vi "Start Module.vi"(6 "Show Main VI Diagram on Init (F)":bool, 7 "Panel":refnum<class "Panel.lvclass"> caption="Panel (Window)", 8 "error in (no error)":errorcluster) -> (0 "error out":errorcluster, 1 "Wait for Event Sync?":bool, 2 "Chart Broadcast Events":T1, 3 "Module Was Already Running?":bool, 4 "Module Name":string)   [LabVIEW 2024, in "Chart.lvlib"]
doc: "Launches the Module Main.vi.\n_____\nCreated using DQMH Event Scripter 6.0.0.122.\n\n<b>Note:</b> This VI was modified by the <b>Validate DQMH Module</b> tool to add calls to the Semaphore VIs to synchronize actions between the Start Module and Stop Module VIs.\n\n<b>Note:</b> This VI was modified by the <b>Validate DQMH Module</b> tool to add the 'Show Main VI Diagram on Init' functionality included in DQMH 6.1.\n\nThe <b>Validate DQMH Module</b> tool added a 'Module Name' output to this VI."
uses:
  Chart.lvlib
  Broadcast Events--cluster.ctl
  Did Init Argument--cluster.ctl
  Status Updated Argument--cluster.ctl
  Error Reported Argument--cluster.ctl
  Stop Argument--cluster.ctl
  Get Module Execution Status Argument--cluster.ctl
  <vilib>/MGI/Panel Manager/Panel/Panel/Panel.lvclass
  <vilib>/Delacor/Delacor QMH/Libraries/Module Admin_class/Delacor_lib_QMH_Module Admin.lvclass
  <vilib>/Delacor/Delacor QMH/Libraries/Module Admin_class/Delacor_lib_QMH_Module Admin.lvclass/Delacor_lib_QMH_Module Admin.ctl
  <vilib>/Delacor/Delacor QMH/Libraries/Module Admin_class/Delacor_lib_QMH_Set External Launch.vi
  <vilib>/MGI/Panel Manager/Panel/Panel/Window/Window.lvclass
  C:/Program Files/National Instruments/LabVIEW 2025/vi.lib/MGI/Panel Manager/Panel/Panel/Panel.lvclass
  <vilib>/MGI/Panel Manager/Panel/Panel/Window/Window.vi
  <vilib>/Utility/error.llb/Error Cluster From Error Code.vi
  <vilib>/ErrorRing/Error Ring.xnode
  <vilib>/MGI/Panel Manager/Panel/Panel.lvlib
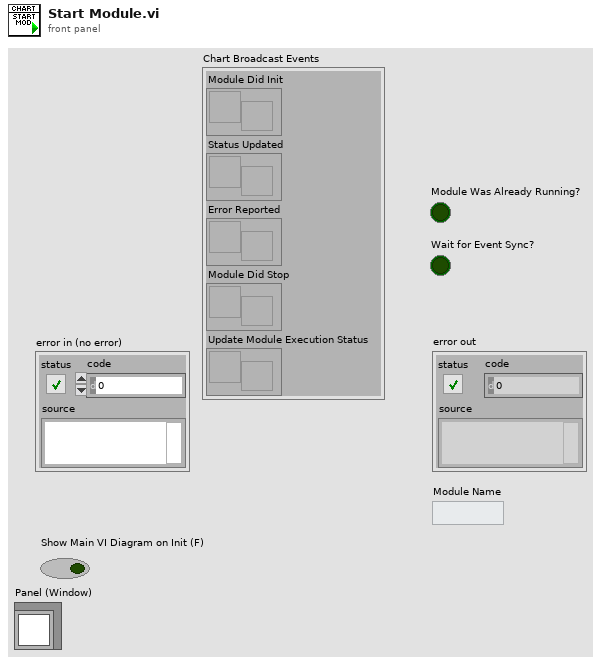
[diagram p1: front panel]
types:
  T1 = typedef "Chart.lvlib/Broadcast Events--cluster.ctl" = cluster{"Module Did Init":refnum<user-event>, "Status Updated":refnum<user-event>, "Error Reported":refnum<user-event>, "Module Did Stop":refnum<user-event>, "Update Module Execution Status":refnum<user-event>}
  T2 = enum32{"Bad", "Idle", "Run top level", "Running"}
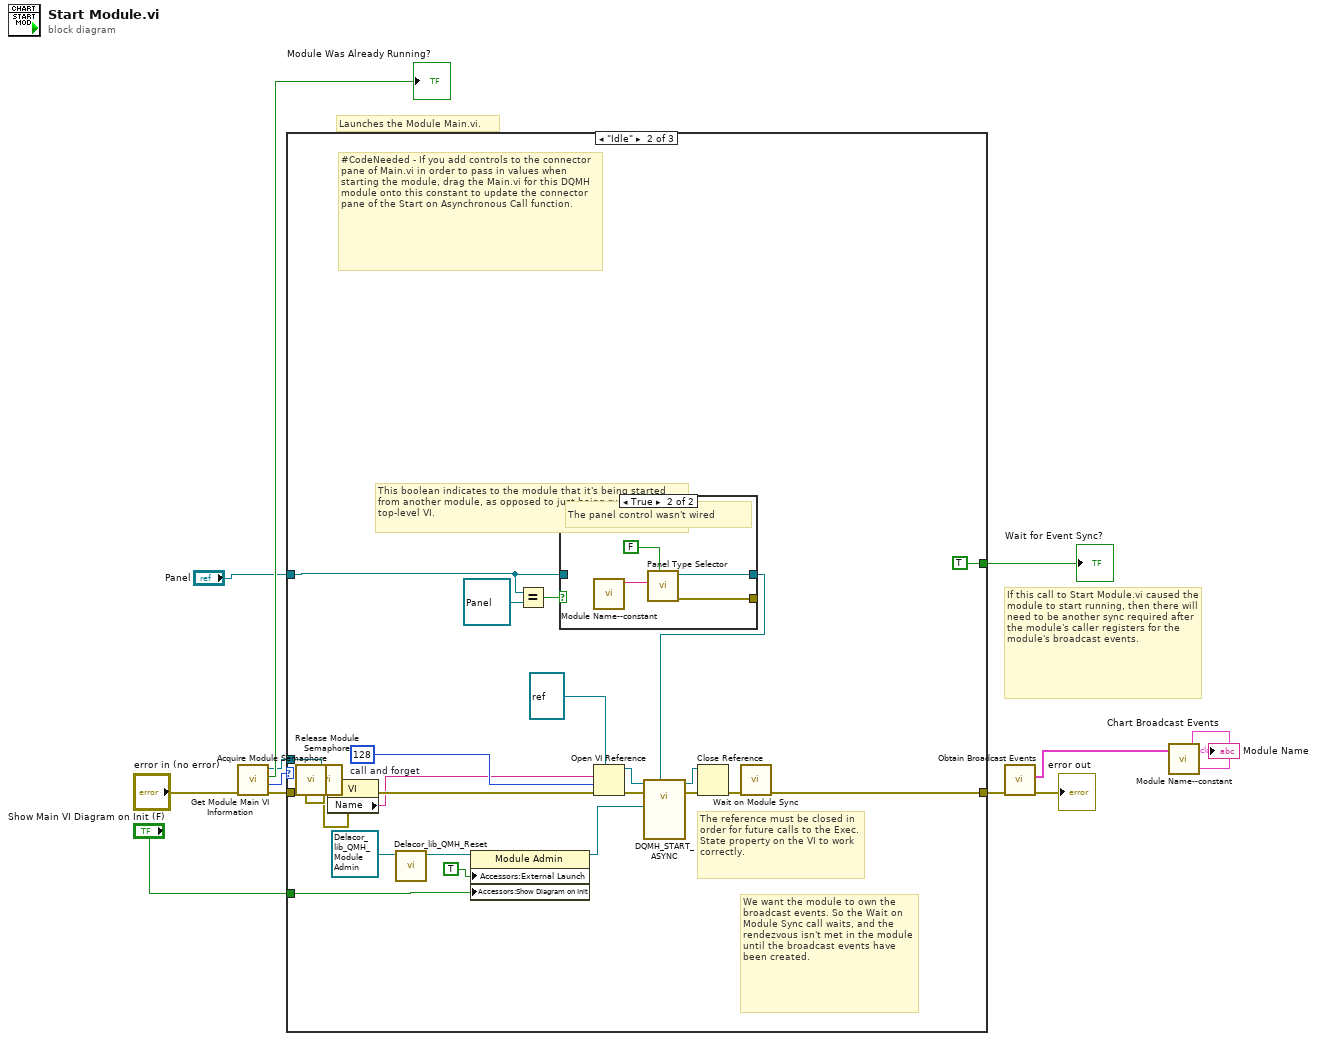
[diagram p0: block diagram]
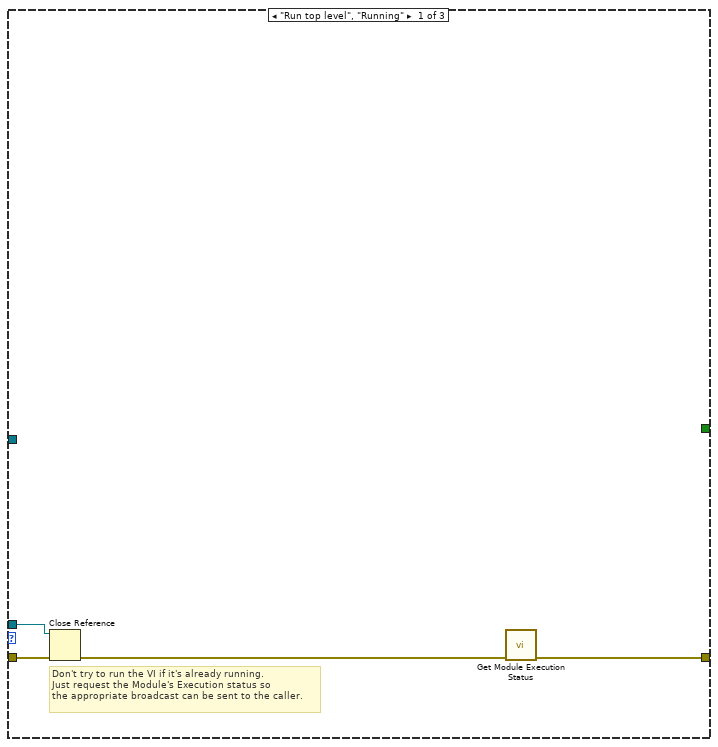
[diagram p2: hidden frame]
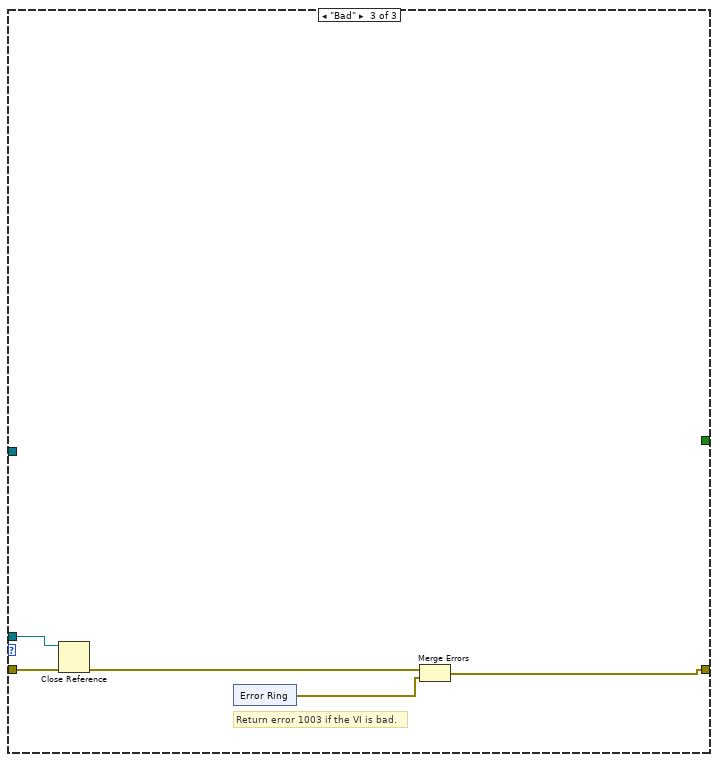
[diagram p4: hidden frame]
diagram:
  # "If this call to Start Module.vi caused the module to start running, then there will need to be another sync required after the module's caller registers for the module's broadcast events."
  # "Launches the Module Main.vi."
  n1 = call "Get Module Main VI Information.vi"("error in (no error)"="error in (no error)") -> ("error out"=w10:errorcluster, "Execution State"=w9:T2, "Is Module Running?"=→"Module Was Already Running?":bool, "Module Main VI"=w7:refnum<vi>)  [unwired: 7 in]
  n2 = case shown="\"Idle\"" w9 {
    tunnel: w10 -> [w16 w40 w50]
    tunnel: w7 -> [w15 w35 w49]
    tunnel: [w13 w25 w47] -> w6
    tunnel: [_ TRUE _] -> w12
    tunnel: "Panel" -> [_ w21 _]
    tunnel: "Show Main VI Diagram on Init (F)" -> [_ w17 _]
    frame "Run top level", "Running" {
      # "Don't try to run the VI if it's already running.\nJust request the Module's Execution status so\nthe appropriate broadcast can be sent to the caller."
      n3 = Close Reference(reference=w15, error in (no error)=w16) -> (error out=w14:errorcluster)
      n4 = call "Get Module Execution Status.vi"("error in (no error)"=w14) -> ("error out"=w13:errorcluster)  [unwired: 10 in]
    }
    frame "Idle" {
      w32 = 128  # call and forget
      # "#CodeNeeded - If you add controls to the connector pane of Main.vi in order to pass in values when starting the module, drag the Main.vi for this DQMH module onto this constant to update the connector pane of the Start on Asynchronous Call function."
      # "The reference must be closed in order for future calls to the Exec.State property on the VI to work correctly."
      # "We want the module to own the broadcast events. So the Wait on Module Sync call waits, and the rendezvous isn't met in the module until the broadcast events have been created."
      # "This boolean indicates to the module that it's being started from another module, as opposed to just being run as a top-level VI."
      n5 = call "Acquire Module Semaphore.vi"("error in"=w40) -> ("error out"=w19:errorcluster)  [unwired: 10 in]
      n6 = call "Release Module Semaphore.vi"("error in"=w19) -> ("error out"=w18:errorcluster)  [unwired: 10 in]
      n7 = property class="VI"(reference=w35, error in=w18) -> (error out=w34:errorcluster, "Name"=w27:string)  [unwired: 1 out]
      n8 = call-dynamic "Delacor_lib_QMH_Reset.vi"("Mod Admin in"=refnum<class "Delacor_lib_QMH_Module Admin.lvclass"> refnum) -> ("Mod Admin out"=w38:refnum<class "Delacor_lib_QMH_Module Admin.lvclass">)  [unwired: 9 in, 1 out]
      n9 = property on="DQMH_ADMIN_PROP_NODE" class="Module Admin"(reference=w38, "Accessors:External Launch"=TRUE ("DQMH_EXTERNAL_LAUNCH"), "Accessors:Show Diagram on Init"=w17) -> (reference out=w24:refnum<class "Delacor_lib_QMH_Module Admin.lvclass">)  [unwired: 1 in, 1 out]
      n10 = Equal?(x=w21, y=refnum<class "Panel.lvclass"> refnum) -> (x = y?=w22:bool)
      n11 = case shown="True" w22 {
        tunnel: w21 -> [w41 _]
        tunnel: [w41 w45] -> w20
        tunnel: [_ w42] -> _
        frame False {
          # "A panel object was wired in."
        }
        frame True {
          # "The panel control wasn't wired"
          n12 = call "Module Name--constant.vi"() -> ("Module Name"=w43:string)  [unwired: 11 in]
          n13 = call-poly <vilib>:"Panel Type Selector.vi"("Autoshow? (T)"=FALSE, "Default Title"=w43) -> ("error out"=w42:errorcluster, "Window out"=w45:refnum<class "Window.lvclass">)  [unwired: 8 in]
        }
      }
      n14 = Open VI Reference(type specifier VI Refnum (for type only)=refnum<vi> refnum ("DQMH_TYPE_SPECIFIER"), vi path=w27, options=w32, error in (no error)=w34) -> (vi reference=w30:refnum<vi>, error out=w31:errorcluster)  [unwired: 2 in]
      n15 = call-by-ref "DQMH_START_ASYNC"(reference=w30, error in=w31, "Panel"=w20, "Module Admin"=w24) -> (reference out=w28:refnum<vi>, error out=w29:errorcluster)  [unwired: 10 in]
      n16 = Close Reference ("DQMH_CLOSE_REF")(reference=w28, error in (no error)=w29) -> (error out=w26:errorcluster)
      n17 = call "Wait on Module Sync.vi"("error in (no error)"=w26) -> ("error out"=w25:errorcluster)  [unwired: 10 in]
    }
    frame "Bad" {
      # "Return error 1003 if the VI is bad."
      n18 = Close Reference(reference=w49, error in (no error)=w50) -> (error out=w48:errorcluster)
      n19 = xnode "Error Ring"() -> ("error out"=w46:errorcluster)
      n20 = Merge Errors(w48, w46) -> (w47:errorcluster)
    }
  }
  "Wait for Event Sync?" <- w12
  n21 = call "Obtain Broadcast Events.vi"("error in (no error)"=w6) -> ("error out"=→"error out":errorcluster, "Chart Broadcast Events"=→"Chart Broadcast Events":T1)  [unwired: 9 in]
  n22 = call "Module Name--constant.vi"() -> ("Module Name"=→"Module Name":string)  [unwired: 11 in]
